vi "Write Configuration.vi"(8 "error in (no error)":errorcluster, 10 "Configuration":T1, 11 "RandomNumberLogger Controller in":refnum<class "RandomNumberLogger Controller.lvclass">) -> (0 "error out":errorcluster, 3 "RandomNumberLogger Controller out":refnum<class "RandomNumberLogger Controller.lvclass">)   [LabVIEW 2020, in "RandomNumberLogger.lvlib" / "RandomNumberLogger Controller.lvclass"]
doc: "<b>Write Configuration</b>\nWrites the configuration information to the plugin controller class data."
uses:
  RandomNumberLogger Controller.lvclass
  RandomNumberLogger Controller.lvclass/RandomNumberLogger Controller.ctl
  PE/Configuration.ctl
  PE/RandomNumberLogger.lvclass
panel:
  # "#via_ignore"
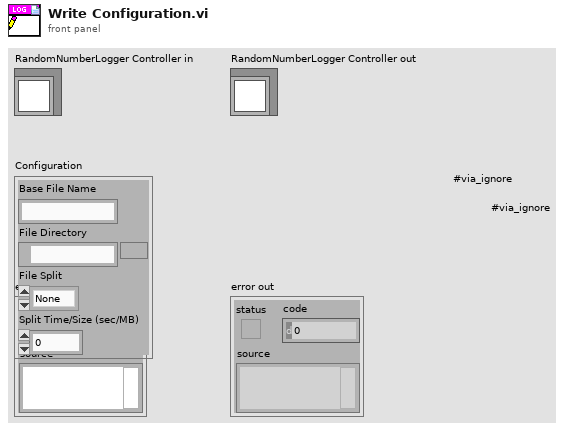
[diagram p1: front panel]
types:
  T1 = typedef "RandomNumberLogger.lvlib/RandomNumberLogger.lvclass/Configuration.ctl" = cluster{"Base File Name":string, "File Directory":path, "File Split":enum16{"None", "Time", "Size"}, "Split Time/Size (sec/MB)":dbl}
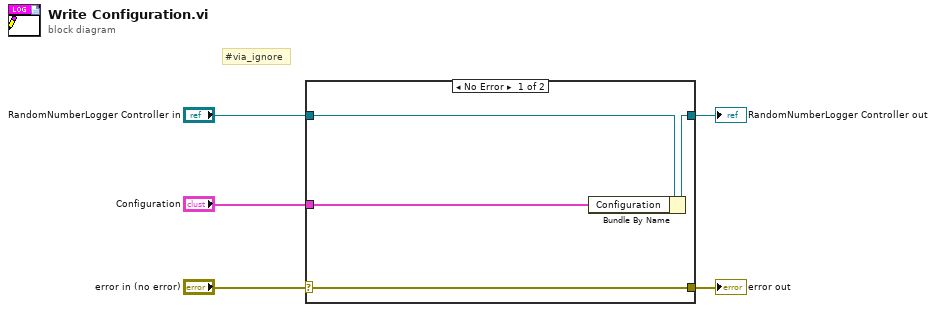
[diagram p0: block diagram]
diagram:
  # "#via_ignore"
  n1 = case shown="No Error" "error in (no error)" {
    selector: "error in (no error)" -> [w9 w10]
    tunnel: [w9 w10] -> w4
    tunnel: [w7 w11] -> w2
    tunnel: "RandomNumberLogger Controller in" -> [w8 w11]
    tunnel: "Configuration" -> [w6 _]
    frame No Error {
      n2 = Bundle By Name(cluster=w8, "Configuration"=w6) -> (w7:refnum<class "RandomNumberLogger Controller.lvclass">)
    }
    frame Error {
    }
  }
  "error out" <- w4
  "RandomNumberLogger Controller out" <- w2
